vi "Extract 2 Cols into 2-col array.vi"(9 "Column 2 Index":i32, 10 "Array in":dbl[][][](array[numeric]), 11 "Column 1 Index":i32) -> (3 "Array out":dbl[][](array[numeric]))   [LabVIEW 2011]
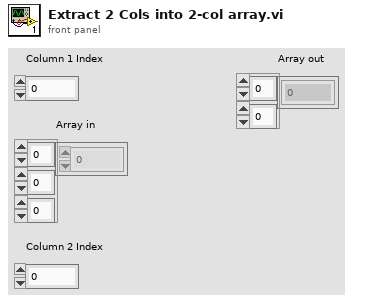
[diagram p1: front panel]
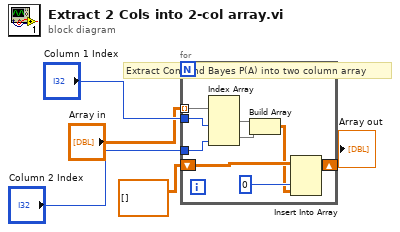
[diagram p0: block diagram]
diagram:
  n1 = for {
    tunnel: "Array in" -> [w14] mode=indexing
    shift-right: [w10] -> w2
    shift-left: dbl[][] [] -> [w13]
    tunnel: "Column 1 Index" -> [w7]
    tunnel: "Column 2 Index" -> [w6]
    # "Extract Conf and Bayes P(A) into two column array"
    n2 = Index Array(array=w14, index (col) #1=w7, index (col) #2=w6) -> (element #1=w8:dbl[], element #2=w9:dbl[])  [unwired: 2 in]
    n3 = Build Array(w8, w9) -> (w11:dbl[][])
    n4 = Insert Into Array(array=w13, index (col)=0 ("disabled index (col)"), new element=w11) -> (w10:dbl[][])  [unwired: 1 in]
  }
  "Array out" <- w2
